vi "CAN open.vi"(4 "error in (no error)":errorcluster, 7 "CANopen in":refnum<class "CANopen.lvclass">) -> (0 "error out":errorcluster, 3 "CANopen out":refnum<class "CANopen.lvclass">)   [LabVIEW 2024]
doc: "Establishes a connection with the CAN bus using the given parameters."
uses:
  CANopen.lvclass/CANopen.ctl
  <resource>/objmgr/xnet.rc
  <vilib>/xnet/xnet.llb/XNET Create Session (Frame Input Stream).vi
  CANopen.lvclass
panel:
  out "Interface:CAN:Termination":u32(ring) items=["Off", "On"]
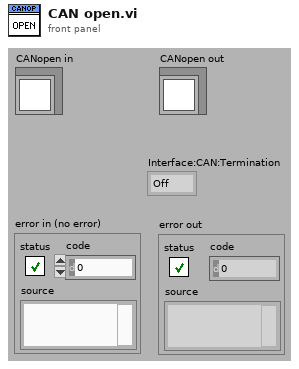
[diagram p1: front panel]
types:
  T1 = typedef "LVStringsAndValuesArrayTypeDef_U32.ctl" = cluster{"String":string, "Value":u32}[]
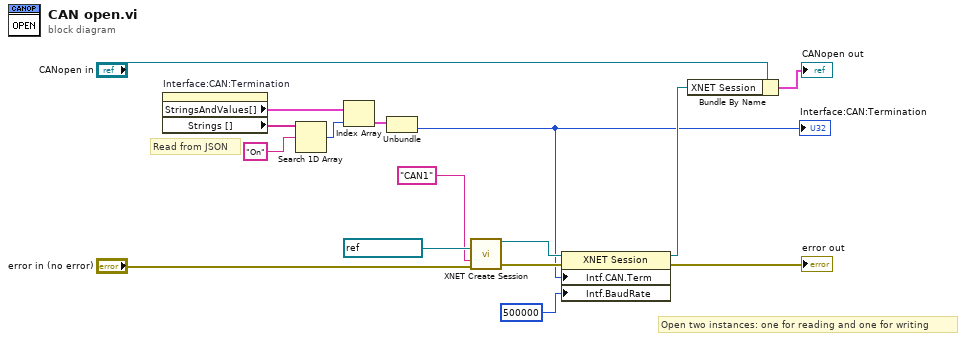
[diagram p0: block diagram]
diagram:
  # "Read from JSON"
  # "Open two instances: one for reading and one for writing"
  n1 = property on="Interface:CAN:Termination" class="Ring (strict)"() -> ("StringsAndValues[]"=w7:T1, "Strings []"=w8:string[])  [unwired: 2 in, 2 out]
  n2 = Search 1D Array(1D array=w8, element="On") -> (index of element=w6:i32)  [unwired: 1 in]
  n3 = Index Array(array=w7, index=w6) -> (element=w5:cluster{"String":string, "Value":u32})
  n4 = Unbundle(w5) -> ("Value"=w4:u32)  [unwired: 1 out]
  "Interface:CAN:Termination" <- w4
  n5 = call-poly <vilib>:"XNET Create Session.vi"("cluster (:memory:)"=refnum<k21> ":memory:" ("CAN Cluster"), "interface"="CAN1" ("element"), "error in (no error)"="error in (no error)") -> ("session out"=w13:refnum<k21>, "error out"=w14:errorcluster)  [unwired: 11 out]
  n6 = property class="XNET Session"(reference=w13, error in=w14, "Intf.CAN.Term"=w4, "Intf.BaudRate"=u32 500000 ("Interface:Baud Rate")) -> (reference out=w10:refnum<k21>, error out=→"error out":errorcluster)
  n7 = Bundle By Name(cluster="CANopen in", "XNET Session"=w10) -> (→"CANopen out":cluster{})
